vi "AlliGator FLI Dataset Loading Core.vi"(4 "Data Description":string, 5 "Control References":T4, 6 "Metadata":string, 7 "Image Type":string, 8 "error in (no error)":errorcluster, 9 "FLI Data File Information":T1, 10 "selected path":path, 11 "Data Value Reference in":refnum<data-value>) -> (0 "error out":errorcluster, 2 "Message":string, 3 "Data Value Reference out":refnum<data-value>)   [LabVIEW 2021, in "AlliGator Files.lvlib"]
doc: "Core VI handling loading the multiple gate images of a dataset as well as associated information and metadata. It dynamically calls a dataset-specific set of VIs to perform the actual loading."
uses:
  AlliGator Files.lvlib
  GUI/AlliGator Dataset Ctrl Refnums.ctl
  Source Image/AlliGator Displayed Image.ctl
  HDF5/AlliGator FLI Data File Information.ctl
  Phasor/Phasor Fluorescence Lifetime Parameters v3.ctl
  AlliGator FLI Dataset Type.ctl
  Internal Variables/AlliGator Internal Variables v2.ctl
  <vilib>/vision/Image Controls.llb/IMAQ Image.ctl
  Internal Variables/AlliGator Gate Image Set.ctl
  AlliGator Data Series Type.ctl
  Dual-Channel Datasets/AlliGator Dataset Channel.ctl
  Settings/AlliGator Gate Arithmetic.ctl
  Image/Named ROI Description.ctl
  Phasor Graph/AlliGator Decay Metadata v3.ctl
  Decay Analysis/Decay Preprocessing/AlliGator Decay Background Subtraction Info.ctl
  Decay Analysis/Decay Preprocessing/AlliGator Baseline Subtraction Method.ctl
  Graphs/XY Graph/XY Graph Plot Shift Parameters.ctl
  Graphs/XY Graph/XY Graph Plot Shift Method.ctl
  Decay Analysis/Decay Preprocessing/AlliGator Decay Extrapolation Parameters.ctl
  Phasor/Calibration Phasor (m, phi).ctl
  Phasor/Phasor Reference Series.ctl
  Phasor/Phasor Calibration Map v2.ctl
  Phasor/Phasor (g, s).ctl
  Phasor Graph/AlliGator Raw Phasor Plot Data v5.ctl
  Phasor/Phasor Standard Deviation Options.ctl
  Phasor Plot/AlliGator Phasor Multi-Harmonic Data.ctl
  Phasor/Phasor Harmonic Data.ctl
  Decay Fit Parameter Map/AlliGator Decay Fit Options & Parameters v4.ctl
  Fits/IRF(X)PSED/Decay Fit Options v4.ctl
  Fits/Decay Convolution/Decay Model.ctl
  Fits/Residual Type.ctl
  Fits/IRF(X)PSED/Fit Weights Type v2.ctl
  Fits/Non-linear Fitting Method v2.ctl
  Fits/Fit Calculation Method.ctl
  Fits/Non-linear Fitting Algorithm.ctl
  Decay Analysis/Decay Fit/AlliGator Decay Fit Parameter Constraints 2.ctl
  Fits/IRF(X)PSED/Decay Fit Parameters In List.ctl
  Fits/IRF(X)PSED/MLE Baseline Offset Type.ctl
  Decay Analysis/Decay Preprocessing/AlliGator Decay Preprocessing Parameters.ctl
  Fits/IRF(X)PSED/Decay Fit Parameters & Derived Quantities List v2.ctl
  Fits/IRF(X)PSED/Decay Fit Result Constraint.ctl
  Decay Fit Parameter Map/AlliGator Parameter Maps Data.ctl
  AlliGator Image Pre-processing Parameters.ctl
  Arrays/Kernel Type.ctl
  Arrays/Smoothing Algorithm.ctl
  SwissSPAD/SwissSPAD Live_Image Display Options.ctl
  AlliGator Image Pre-processing Step.ctl
  HDF5/AlliGator FLI Image Stack Action.ctl
  Globals, Variables, Constants/AlliGator Variables List.ctl
  AlliGator After Loading Dataset Information.ctl
  AlliGator ICCD-specific Information.ctl
  Globals, Variables, Constants/AlliGator Abort.vi
  <vilib>/Utility/error.llb/Error Cluster From Error Code.vi
  <vilib>/ErrorRing/Error Ring.xnode
  Source Image/AlliGator Source Image.lvlib
  HDF5/AlliGator HDF5.lvlib
  Time/Time.lvlib
  Arrays/Arrays.lvlib
  Strings/Strings.lvlib
  GUI/AlliGator GUI.lvlib
  GUI/GUI.lvlib
  Error/Error.lvlib
  Dual-Channel Datasets/AlliGator Dual-Channel Datasets.lvlib
  Image/Image.lvlib
  SwissSPAD/SwissSPAD Live.lvlib
  Globals, Variables, Constants/AlliGator Globals, Variables & Constants.lvlib
  Files/Files.lvlib
  Phasor/Phasor.lvlib
  Decay Analysis/Decay Preprocessing/AlliGator Decay Preprocessing.lvlib
  Graphs/XY Graph/XY Graph Add-Ons.lvlib
  Phasor Graph/AlliGator Phasor Graph.lvlib
  Phasor Plot/AlliGator Phasor Plot.lvlib
  Fits/Fits.lvlib
  Decay Analysis/Decay Fit/AlliGator Decay Fit.lvlib
  Internal Variables/AlliGator Internal Variables.lvlib
  Settings/AlliGator Settings.lvlib
  Decay Fit Parameter Map/AlliGator Decay Fit Parameter Map.lvlib
panel:
  out "Dual-Channel Dataset":bool
  out "# created images":i32
  out "# Disposed Images":i32
  # "see the AlliGator License on the block diagram (Ctrl+E or Window:Show Block Diagram)"
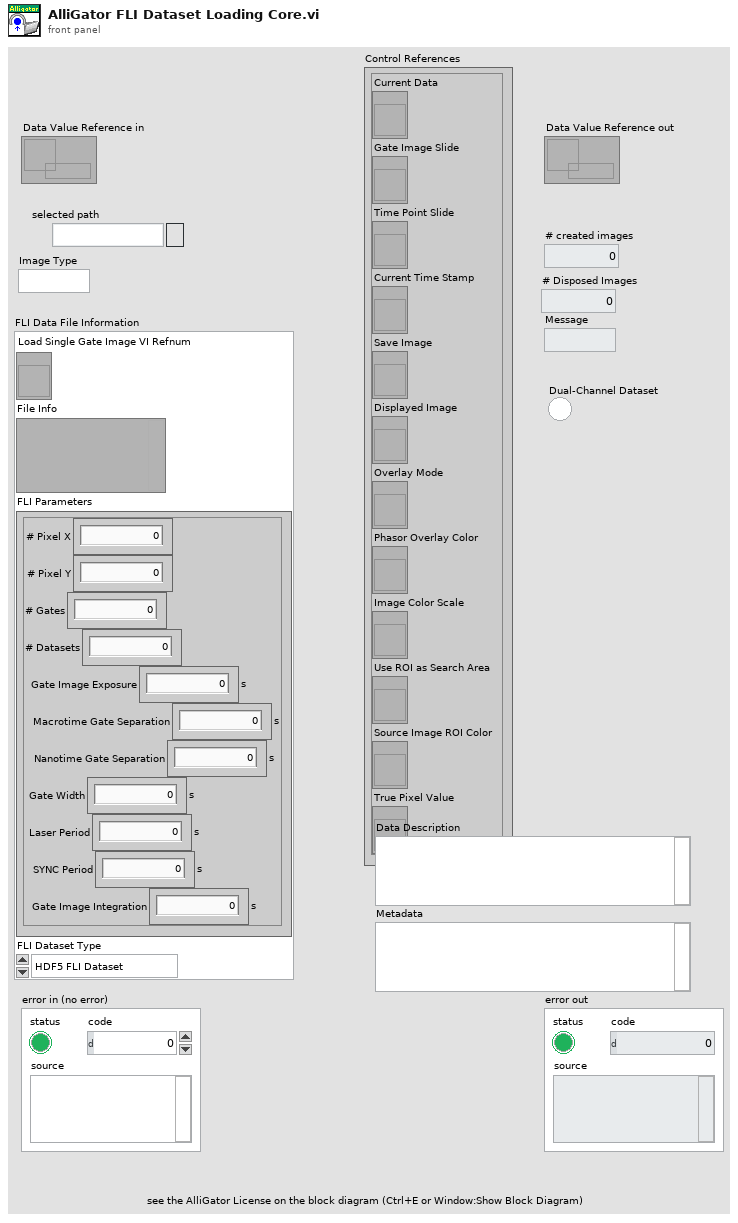
[diagram p1: front panel]
types:
  T1 = typedef "AlliGator HDF5.lvlib/AlliGator FLI Data File Information.ctl" = cluster{"Load Single Gate Image VI Refnum":refnum<vi>, "File Info":variant, "FLI Parameters":T2, "FLI Dataset Type":T3}
  T2 = typedef "Phasor.lvlib/Phasor Fluorescence Lifetime Parameters v3.ctl" = cluster{"# Pixel X":i32, "# Pixel Y":i32, "# Gates":i32, "# Datasets":i32, "Gate Image Exposure":dbl[unit], "Macrotime Gate Separation":dbl[unit], "Nanotime Gate Separation":dbl[unit], "Gate Width":dbl[unit], "Laser Period":dbl[unit], "SYNC Period":dbl[unit], "Gate Image Integration":dbl[unit]}
  T3 = typedef "AlliGator Files.lvlib/AlliGator FLI Dataset Type.ctl" = enum16{"HDF5 FLI Dataset", "Gate Image Folder", ".sdt FLI Dataset (Becker & Hickl)", ".ptu FLI Dataset (PicoQuant)", "SS1 FLI Dataset", "SS2 FLI Dataset", "I/m/phi Dataset", ".bin FLI Dataset (PicoQuant Binned)", ".bin FLI Dataset (Piccolo Binned)", ".mat FLI Dataset"}
  T4 = typedef "AlliGator GUI.lvlib/AlliGator Dataset Ctrl Refnums.ctl" = cluster{"Current Data":refnum<vi>, "Gate Image Slide":refnum<vi>, "Time Point Slide":refnum<vi>, "Current Time Stamp":refnum<vi>, "Save Image":refnum<vi>, "Displayed Image":refnum<vi>, "Overlay Mode":refnum<vi>, "Phasor Overlay Color":refnum<vi>, "Image Color Scale":refnum<vi>, "Use ROI as Search Area":refnum<vi>, "Source Image ROI Color":refnum<vi>, "True Pixel Value":refnum<vi>}
  T5 = typedef "AlliGator Files.lvlib/AlliGator Image Pre-processing Parameters.ctl" = cluster{"Pile-up Correction":bool, "Pixel Well Capacity":u32, "Use Image Binning":bool, "X Bin":i32, "Y Bin":i32, "Use Image Smoothing":bool, "Kernel Type":T6, "Bin":i32, "Algorithm":T7, "Hot Pixel Removal":T8, "Dataset Scaling Factor":dbl, "Image Pre-processing Steps":T9[]}
  T6 = typedef "Arrays.lvlib/Kernel Type.ctl" = enum16{"Uniform", "Bilinear", "Gaussian"}
  T7 = typedef "Arrays.lvlib/Smoothing Algorithm.ctl" = enum16{"Rapid", "Thorough"}
  T8 = typedef "SwissSPAD Live.lvlib/SwissSPAD Live_Image Display Options.ctl" = cluster{"Remove Screamers":bool, "Delta":sgl, "Equalize Histogram":bool, "Percentile":sgl, "Hot Pixel Mask Image":path, "Use Hot Pixel Mask":bool}
  T9 = typedef "AlliGator Files.lvlib/AlliGator Image Pre-processing Step.ctl" = enum16{"Remove Screamers", "Pile-up Correction", "Binning", "Smoothing", "Rescaling", "Dead Left Column Correction"}
  T10 = typedef "AlliGator Source Image.lvlib/AlliGator Image Loading Options.ctl" = cluster{"Pixel Well Capacity":u32, "Pile-up Correction":bool, "Gate Step":i32, "Image Smoothing Options":T11, "Gates to Skip":T12, "File Background Subtraction":bool, "Background File Path":path, "Image Binning Options":T13, "# Gates":u32, "Gates to Keep":T14, "Define Gates to":bool, "Hot Pixel Removal":T8, "Dataset Scaling Factor":dbl, "Image Pre-processing Steps":T9[]}
  T11 = typedef "AlliGator Settings.lvlib/AlliGator Image Smoothing Options.ctl" = cluster{"Use Image Smoothing":bool, "Kernel Type":T6, "Bin":i32, "Algorithm":T7}
  T12 = typedef "AlliGator Settings.lvlib/AlliGator Background Subtraction Parameters.ctl" = cluster{"Start":u32, "End":u32}
  T13 = typedef "AlliGator Source Image.lvlib/AlliGator Image Binning Options.ctl" = cluster{"Use Image Binning":bool, "X Bin":i32, "Y Bin":i32}
  T14 = typedef "AlliGator Settings.lvlib/AlliGator Gates to Keep.ctl" = cluster{"First":u32, "Last":u32}
  T15 = typedef "AlliGator Settings.lvlib/AlliGator Gate Arithmetic.ctl" = enum16{"None", "INT-G2", "G2/INT*<INT>", "(1 - G2/INT)*<INT>"}
  T16 = typedef "AlliGator Dual-Channel Datasets.lvlib/AlliGator Dataset Channel.ctl" = enum16{"G2", "INT"}
  T17 = typedef "Image.lvlib/Image Characteristics.ctl" = cluster{"Calibration":T18, "File Type":string, "X Resolution":i32, "Y Resolution":i32, "File Data Type":i32, "Image Type":T20}
  T18 = typedef "Simple Grid Descriptor" = cluster{"X Step":sgl, "Y Step":sgl, "Unit":T19}
  T19 = typedef "Image Unit" = enum32{"Undefined", "Angström", "Micrometer", "Millimeter", "Centimeter", "Meter", "Kilometer", "Microinch", "Inch", "Feet", "Nautical miles", "Standard miles", "Steps"}
  T20 = typedef "Image Type" = u32
  T21 = typedef "AlliGator HDF5.lvlib/AlliGator FLI Image Stack Action.ctl" = enum16{"Init", "Get Image", "Close"}
  T22 = typedef "AlliGator Globals, Variables & Constants.lvlib/AlliGator Variables List.ctl" = enum16{"---- GUI ----", "GUI:Initialization Status", "GUI:State Indicators Refnum", "GUI:Original AlliGator Menu Items", "GUI:Current Action Loop State", "GUI:Script in progress", "GUI:Playback", "GUI:Loop Playback", "GUI:Search ROI Used", "GUI:Search ROI", "Decay Graph Max Legend Size", "Intensity Graph Max Legend Size", "Decay Statistics Graph Max Legend Size", "Phasor Graph Max Legend Size", "Phasor Ratio Graph Max Legend Size", "Lifetime Graph Max Legend Size", "---- Files ----", "Files:Export Dataset Frames as Individual Files", "Files:Show Batch Export Help Balloons", "Files:Frames in Dataset", "Files:ptu File Frame Start Indices", "Files:Current Frame in Dataset", "Files:Current Frame Timestamp", "Files:Dataset Loaded", "Files:Dataset Metadata", "Files:Dataset Channel", "Files:Dataset Data Description", "Files:Background Dataset Metadata", "Files:Background Dataset Channel", "Files:Background Dataset Data Description", "Files:Background File Subtraction", "Files:Background File Path", "Files:Background File Pile-up Correction", "Files:Background File Pixel Well Capacity", "Files:Background File Scaling Factor", "Files:Current Dataset Load Settings", "Files:Dataset Path", "Files:ICCD-specific Information", "Files:Macrotime Gate Separation", "------ Python Plugins ------", "Python Plugins:Information", "Python Plugins:Python Session", "Python Plugins:Valid Python Session?", "---- Source Image ----", "Source Image:ROIs", "Source Image:Current ROI", "Source Image:ROI Event Refnum", "X_Source Image:Display Range", "X_Source Image:Palette Information", "X_Source Image:Type of Displayed Image", "X_Time Gate Slider", "Source Image:Palette List", "Source Image:Scale", "Source Image:ROI Overlay Color", "Source Image:Overlay to Erase", "Source Image:Is Displayed Image Accumulated", "Source Image:White Light Image Modified", "Source Image:Mask Image Modified", "---- Image Profile Window ----", "Image Profile:Window Event Refnum", "Image Profile:IntensityType", "Image Profile:Intensity Average Type", "Image Profile:Intensity-weighted SDV", "Image Profile:Box Profile Type", "Image Profile:Window Open", "Image Profile:Plotted Fit Parameter", "------ Phasor Graph -------", "Phasor Graph:Show Line", "---- Phasor Plot ---", "Phasor Plot:Parameters Changed", "Phasor Plot:FLI Dataset Modified since last Calculation", "Phasor Harmonics Data", "Selected Phasor Harmonics", "Phasor Harmonic Manager Event Refnum", "Phasor Plot:ROIs", "Phasor Plot:Current ROI", "Phasor Plot:ROI Event Refnum", "Phasor Plot:Image Reference Points", "Phasor Plot:Computed", "Phasor Plot:Palette Information", "Phasor Plot:Palette List", "Phasor Plot:Phasor Ratio Palette Information", "Phasor Plot:Phasor Ratio Palette List", "Phasor Plot:Image Scale", "Phasor Plot:Image Overlay to Erase", "Phasor Plot:Image Elements to Update", "Phasor Plot:Current Calculation Parameters", "Phasor Plot:Current Calibration Options", "Phasor Plot:Reset Cumulated Phasor Plot", "Phasor Plot:Reference 1", "Phasor Plot:Lifetime Reference 1", "Phasor Plot:Reference 1 Frequency", "Phasor Plot:Reference 2", "Phasor Plot:Lifetime Reference 2", "Phasor Plot:Reference 2 Frequency", "---- Decay Analysis ----", "Number of Selected Decays to Fit", "LS Fit Results", "LAR Fit Results", "BS Fit Results", "Last Decay Max - Min", "Best Fit Parameters", "Best Fit Parameter Names", "Actual Size X", "Actual Size Y", "Binning X", "Binning Y", "Actual # Gates", "Dataset Number", "Gates to...", "Gates Skipped", "Gates to keep", "Gate Step", "Gate Separation", "Reversed Gates", "Pile-up Correction", "Pixel Well Capacity", "Background Subtracted", "Background Subtraction Method", "Background Definition Range", "Background File (deprecated)", "Number of Dataset Accumulated", "Array of Accumulated Dataset Paths", "Do Averaged Datasets", "Destination File Path", "Process Plot Target", "Use 1/D as Phasor Frequency", "---- Decay Fit Parameter Map -----", "Decay Fit Parameter Map:Palette Information", "Decay Fit Parameter Map:Palette List", "Decay Fit Parameter Map:X Resolution", "Decay Fit Parameter Map:Y Resolution", "Decay Fit Parameter Map:Use Decay Fit Result Constraints", "Decay Fit Parameter Map:Decay Fit Result Constraints", "Decay Fit Parameter Map:Decay Fit Result Constraints Applied", "---- Parameter Map ----", "Parameter Map:Palette Information", "Parameter Map:Palette List", "------- Local Decay Window ---------", "Local Decay Graph Window:Event Refnum", "Local Decay Graph Window:Use normalized IRF for convolution", "----- Miscellaneous ----", "Misc:Skippable Dialog Windows Status"}
  T23 = typedef "AlliGator Internal Variables.lvlib/AlliGator Internal Variables v2.ctl" = cluster{"----------------------------- Images -----------------------------":u8, "Displayed Image":T24, "White Light Image":T24, "Mask Image":T24, "ROI Mask Image":T24, "Current Dataset Images 1":T25, "Background Dataset Images 1":T25, "Current Dataset Images 2":T25, "Background Dataset Images 2":T25, "Current Dataset Arithmetic Images":T25, "Accumulated Dataset Images 1":T25, "Accumulated Dataset Images 2":T25, "Accumulated Dataset Arithmetic Images":T25, "----------------------------- File Paths -----------------------------":u8, "Phasor Plot Image":T24, "Decay Fit Parameter Map Image":T24, "Parameter Map Image":T24, "Single Data Point Path":path, "White Light Image Path":path, "Mask Image Path":path, "Time-Series Folder":path, "[Time-Series Paths]":path[], "----------------------------- FLI Dataset -----------------------------":u8, "Current Dataset":i32, "Single Dataset Type":T3, "Current Folder":string, "AlliGator Data Series Type":T26, "# Datasets":i32, "Dual-Channel Dataset":bool, "Selected Channel Name":string, "Dataset Channel":T16, "Channel Arithmetic":T15, "Dual-Channel Background Dataset":bool, "Background Channel":T16, "Dual-Channel Accumulated Dataset":bool, "Start Time":dbl, "[Time-Series Timestamps]":dbl[], "[Intensity Corrections]":dbl[], "Time Series Script":bool, "Type of Displayed Image":T27, "Gate Image Slide":u16, "# Gates":i32, "ROIs":T28[], "----------------------------- Decays -----------------------------":u8, "ROI Decay":cluster{"t Array":dbl[], "I Array":dbl[]}, "Valid Decay":bool, "Decay  Metadata":T30, "Reference Decay Plot Name":string, "Reference Decay":cluster{"t Array":dbl[], "I Array":dbl[]}, "Decay Shift Plot":cluster{"Time Stamps":dbl[], "Decay Shifts":dbl[]}, "[Decays Max Values]":sgl[], "[Decays Min Values]":sgl[], "----------------------------- Calibration -----------------------------":u8, "Calibration Phasor":T36, "Calibration Phasor Series":T37, "Phasor Calibration Map":T38, "Calibration Map MD5 Digest":string, "----------------------------- Phasor Graph -----------------------------":u8, "Last Raw Phasor":T39, "Last Calibrated Phasor":T39, "Last Calibrated Phasor SDV":T39, "Phasor Graph:Phasor Plot":cluster{"g Array":dbl[], "s Array":dbl[]}, "Phasor Graph:Phasor SDV Plot":cluster{"g Array":dbl[], "s Array":dbl[]}, "[Phasor Graph:Raw Phasor Plots]":T40[], "Phasor Plot locked to Ref 1":i32, "[Phasor Plot(s) locked to Ref 1]":i32[], "[Phasor Plot(s) locked to Ref 2]":i32[], "[Pixel Phasors]":T39[], "----------------------------- Phasor Plot -----------------------------":u8, "[[Sum Image]]":dbl[][], "[[CSG Phasors]]":csg[][], "[[Valid Pixel?]]":bool[][], "[[Phasor Ratios]]":dbl[][], "[[Average Lifetimes]]":dbl[][], "Amplitude Weighted Average Lifetime":bool, "I/m/phi Dataset":cluster{"I/m/phi Dataset?":bool, "Base Frequency":dbl[unit], "Harmonic Orders":u8[]}, "Multi Phasor Plot Data":T42, "----------------------------- Decay Fit Parameter Map -----------------------------":u8, "Decay Fit Options & Parameters":T44, "Fit Options: Decay Preprocessing Parameters":T55, "Fit Options: Reference Decay":cluster{"t Array":dbl[], "I Array":dbl[]}, "Is Full Image Parameters Map":bool, "Is Single-Pixels Parameters Map":bool, "NLSF Parameters Map X Resolution":i32, "NLSF Parameters Map Y Resolution":i32, "[Single Decay Fit Parameters]":dbl[], "Fit Model":T46, "[[Multiple Decays Fit Parameters]]":dbl[][], "[[Multiple Decays Fit Parameter SDVs]]":dbl[][], "[[IRFs]]":dbl[][], "[ROI Descriptors]":T29[], "IRF Array Time Axis":dbl[], "Decay Array Time Axis":dbl[], "[Decay Fit Parameter Names]":T56[], "[Decay Sum]":dbl[], "Array of Decay Fit Result Constraints":T57[], "Selected ROIs Array":bool[], "----------------------------- Parameter Maps -----------------------------":u8, "[Map Set Names]":string[], "[Parameter Maps]":T58[], "[[User-defined Quantities]]":dbl[][], "User-defined Quantity":string}
  T24 = typedef "IMAQ Image.ctl" = refnum<image>
  T25 = typedef "AlliGator Internal Variables.lvlib/AlliGator Gate Image Set.ctl" = cluster{"SGL Image Max":T24, "SGL Image Sum":T24, "SGL Gate Images":T24[], "SGL Image Min":T24}
  T26 = typedef "AlliGator Files.lvlib/AlliGator Data Series Type.ctl" = enum16{"Not a Supported Series", "Gate Images Folder Series", "SwissSPAD 2 Dataset Series", "B&H FLI Dataset Series", "PicoQuant PTU FLI Dataset Series", "PicoQuant BIN FLI Dataset Series", "Piccolo hist BIN FLI Dataset Series", "HDF5 FLI Dataset Series"}
  T27 = typedef "AlliGator Source Image.lvlib/AlliGator Displayed Image.ctl" = enum16{"Single Gate", "Sum of All Gates", "Max of All Gates", "Min of All Gates", "-", "White Ligth Image", "Mask Image"}
  T28 = typedef "Image.lvlib/Named ROI Description.ctl" = cluster{"ROI Descriptor":T29, "ROI Name":string, "Overlay Color":u32}
  T29 = typedef "ROI Descriptor" = cluster{"Global Rectangle":i32[], "Contours":cluster{"ID":enum32{"External", "Internal"}, "Type":u32, "Coordinates":i32[]}[]}
  T30 = typedef "AlliGator Phasor Graph.lvlib/AlliGator Decay Metadata v3.ctl" = cluster{"ROI Descriptor":T29, "ROI Center":cluster{"X":i32, "Y":i32}, "Decay Background Subtraction Info":T31, "Decay Reverted":bool, "Decay Smoothened":bool, "Decay Straightened":bool, "Fitted Tau (Decay Straightening)":dbl, "Decay Shift Parameters":T33, "Decay Shifted":bool, "Decay Extrapolated":bool, "Decay Extrapolation Parameters":T35, "Decay Normalized":bool, "Fold Decay":bool, "# Folds":u32}
  T31 = typedef "AlliGator Decay Preprocessing.lvlib/AlliGator Decay Background Subtraction Info.ctl" = cluster{"Laser Period":dbl[unit], "Gate Duration":dbl[unit], "Baseline Subtraction Method":T32, "Background Definition Range":cluster{"Min Gate":dbl[unit], "Max Gate":dbl[unit]}, "Total Intensity w/o Bkgd Subtraction":dbl, "Bkgd-subtracted Intensity (exp)":dbl, "# Data Points":i32, "Background/Gate":dbl, "Fitted Lifetime":dbl[unit], "Bkgd-subtracted Intensity (theo)":dbl}
  T32 = typedef "AlliGator Decay Preprocessing.lvlib/AlliGator Baseline Subtraction Method.ctl" = enum16{"Mean", "Min", "Square Gated Single-Exponential", "File", "Constant"}
  T33 = typedef "XY Graph Add-Ons.lvlib/XY Graph Plot Shift Parameters.ctl" = cluster{"Type":T34, "Shift":dbl[unit], "Threshold":dbl, "Rotate":bool}
  T34 = typedef "XY Graph Add-Ons.lvlib/XY Graph Plot Shift Method.ctl" = enum16{"Default", "CFD", "Threshold", "Cross-Correlation"}
  T35 = typedef "AlliGator Decay Preprocessing.lvlib/AlliGator Decay Extrapolation Parameters.ctl" = cluster{"Additional Points":u32, "Head Fraction":dbl, "Fitted Tau":dbl, "Use Periodicity":bool, "Use Cursors":bool, "Tail Fraction":dbl}
  T36 = typedef "Phasor.lvlib/Calibration Phasor (m, phi).ctl" = cluster{"m":dbl, "phi":dbl, "Phasor Frequency":dbl[unit], "Reference Lifetime":dbl[unit]}
  T37 = typedef "Phasor.lvlib/Phasor Reference Series.ctl" = cluster{"m Array":dbl[], "phi Array":dbl[], "Phasor Frequency":dbl[unit], "Calibration Lifetime":dbl[unit]}
  T38 = typedef "Phasor.lvlib/Phasor Calibration Map v2.ctl" = cluster{"Phasor Frequency":dbl[unit], "Calibration Lifetime":dbl[unit], "ROI Centers":cluster{"X":i32, "Y":i32}[], "ROI Descriptors":T29[], "Map Resolution X":i32, "Map Resolution Y":i32, "z Array":cdb[]}
  T39 = typedef "Phasor.lvlib/Phasor (g, s).ctl" = cluster{"g":dbl, "s":dbl}
  T40 = typedef "AlliGator Phasor Graph.lvlib/AlliGator Raw Phasor Plot Data v5.ctl" = cluster{"Phasor Plot Name":string, "Raw Phasor Plot":T39[], "Phasor Frequency":dbl[unit], "[Decay Metadata]":T30[], "Raw Phasor Plot SDV":T39[], "Phasor SDV Options":T41, "[Calibration Phasor]":T36[], "Intensity Array":dbl[]}
  T41 = typedef "Phasor.lvlib/Phasor Standard Deviation Options.ctl" = cluster{"Compute Estimated SDV":bool, "# Replicas":u32, "Use Estimated Average Phasor":bool}
  T42 = typedef "AlliGator Phasor Plot.lvlib/AlliGator Phasor Multi-Harmonic Data.ctl" = cluster{"Base Frequency":dbl[unit], "# Harmonics":u8, "Harmonic Orders":u8[], "Phasor Plot Settings Checksum":u64, "Phasor Harmonic Data Array":T43[]}
  T43 = typedef "Phasor.lvlib/Phasor Harmonic Data.ctl" = cluster{"Phasor Harmonic Name":string, "Phasor Plot Settings Checksum":u64, "Phasor Frequency":dbl[unit], "Base Frequency":dbl[unit], "Harmonic Order":u8, "Phasor Plot Parameters":string, "Phasor Array [[CSG]]":csg[][], "Dataset File Path":path}
  T44 = typedef "AlliGator Decay Fit Parameter Map.lvlib/AlliGator Decay Fit Options & Parameters v4.ctl" = cluster{"SYNC Period":dbl[unit], "Fit Options":T45, "Fit Parameter Constraints":T52[], "MLE Baseline Offset":dbl, "MLE Baseline Offset Type":T54}
  T45 = typedef "Fits.lvlib/Decay Fit Options v4.ctl" = cluster{"Show Fit Residuals":bool, "Fit Model":T46, "Residual Type":T47, "Max Decay Percentile":dbl, "Min Decay Percentile":dbl, "Show Full Decay":bool, "Weights":T48, "Fitting Method":T49, "Compute Parameter Uncertainties":bool, "Periodic Boundaries":bool, "Model Calculation":T50, "Period":dbl[unit], "Termination Criteria":cluster{"Max Iterations":i32, "Max Function Calls":i32, "Max Time":dbl[unit], "Function Tolerance":dbl, "Parameter Tolerance":dbl, "Gradient Tolerance":dbl, "Min Lambda":dbl, "Max Lambda":dbl, "Initial Tick Count":u32}, "Offset Resolution":dbl[unit], "Use Local IRF":bool, "Fitting Algorithm":T51, "Show Confidence Interval ":bool, "Confidence Level":dbl}
  T46 = typedef "Fits.lvlib/Decay Model.ctl" = enum16{"1-Exponential", "2-Exponentials"}
  T47 = typedef "Fits.lvlib/Residual Type.ctl" = enum16{"Standard", "Normalized", "Reduced"}
  T48 = typedef "Fits.lvlib/Fit Weights Type v2.ctl" = enum16{"Unweighted", "1/Variance (Neyman)", "1/Variance (Pearson)", "Best of All"}
  T49 = typedef "Fits.lvlib/Non-linear Fitting Method v2.ctl" = enum16{"Least Square", "Least Absolute Residual", "Bisquare", "MLE", "-", "Best of All"}
  T50 = typedef "Fits.lvlib/Fit Calculation Method.ctl" = enum16{"Simulation", "Convolution", "Integration"}
  T51 = typedef "Fits.lvlib/Non-linear Fitting Algorithm.ctl" = enum16{"Levenberg-Marquardt", "Trust-Region Dogleg"}
  T52 = typedef "AlliGator Decay Fit.lvlib/AlliGator Decay Fit Parameter Constraints 2.ctl" = cluster{"Fit Parameter":T53, "Min Value":dbl, "Max Value":dbl, "Global":bool, "Used":bool}
  T53 = typedef "Fits.lvlib/Decay Fit Parameters In List.ctl" = enum16{"Offset", "Baseline", "A_1", "tau_1", "A_2", "tau_2"}
  T54 = typedef "Fits.lvlib/MLE Baseline Offset Type.ctl" = enum32{"Absolute", "Percentage"}
  T55 = typedef "AlliGator Decay Preprocessing.lvlib/AlliGator Decay Preprocessing Parameters.ctl" = cluster{"Background Subtraction":bool, "Straighten Decay":bool, "Reverse Gates":bool, "1-Normalized Decay":bool, "Smoothen Decay":bool, "Smoothing Parameter":dbl, "Shift Decay":bool, "Decay Shift Parameters":T33, "Extrapolate Decay":bool, "Additional Points":u32, "Head Fraction":dbl, "Pixel-Normalize Decay":bool, "Use Periodicity":bool, "Use Cursors":bool, "Tail Fraction":dbl, "Use Decay Pre-Processing":bool, "Fold Decay":bool, "# Folds":u32, "[0-1]-Normalized Decay":bool}
  T56 = typedef "Fits.lvlib/Decay Fit Parameters & Derived Quantities List v2.ctl" = enum16{"Offset", "Baseline", "A_1", "tau_1", "A_2", "tau_2", "<tau>_a", "f1_a", "f2_a", "<tau>_i", "f1_i", "f2_i", "-", "R^2", "Chi^2"}
  T57 = typedef "Fits.lvlib/Decay Fit Result Constraint.ctl" = cluster{"Fit Parameter":enum16{"Offset", "Baseline", "A_1", "tau_1", "A_2", "tau_2", "<tau>_a", "f1_a", "f2_a", "<tau>_i", "f1_i", "f2_i", "-", "R^2", "Chi^2", "Max Relative Residual", "<Residual ACF>", "Residual ACF SDV", "tau_2/tau_1"}, "Min Value":dbl, "Max Value":dbl, "Use Constraint":bool}
  T58 = typedef "AlliGator Decay Fit Parameter Map.lvlib/AlliGator Parameter Maps Data.ctl" = cluster{"Map Set Name":string, "[Parameter Names]":string[], "[[Parameters]]":dbl[][], "[[Parameter SDVs]]":dbl[][], "Decay Array Time Axis":dbl[], "[[IRFs]]":dbl[][], "IRF Array Time Axis":dbl[], "X Resolution":i32, "Y Resolution":i32, "Intensity Array":dbl[]}
  T59 = typedef "AlliGator Files.lvlib/AlliGator ICCD-specific Information.ctl" = cluster{"V MCP":dbl[unit], "X Hardware Binning":dbl, "Y Hardware Binning":dbl, "Gate Image Integration":dbl[unit], "Laser Power":dbl[unit]}
  T60 = typedef "AlliGator Files.lvlib/AlliGator After Loading Dataset Information.ctl" = cluster{"Nanotime Gate Separation":dbl[unit], "Gate Width":dbl[unit], "Laser Period":dbl[unit], "Data Description":string, "# Pixel X":i32, "# Pixel Y":i32, "Gates to Use":cluster{"Start":u32, "End":u32}, "Gate Step":i32, "SYNC Period":dbl[unit], "X Binning":i32, "Y Binning":i32, "Gates to":bool, "Metadata":string, "Gate Image Exposure":dbl[unit], "Gate Image Integration":dbl[unit], "Macrotime Gate Separation":dbl[unit], "ICCD-specific Information":T59}
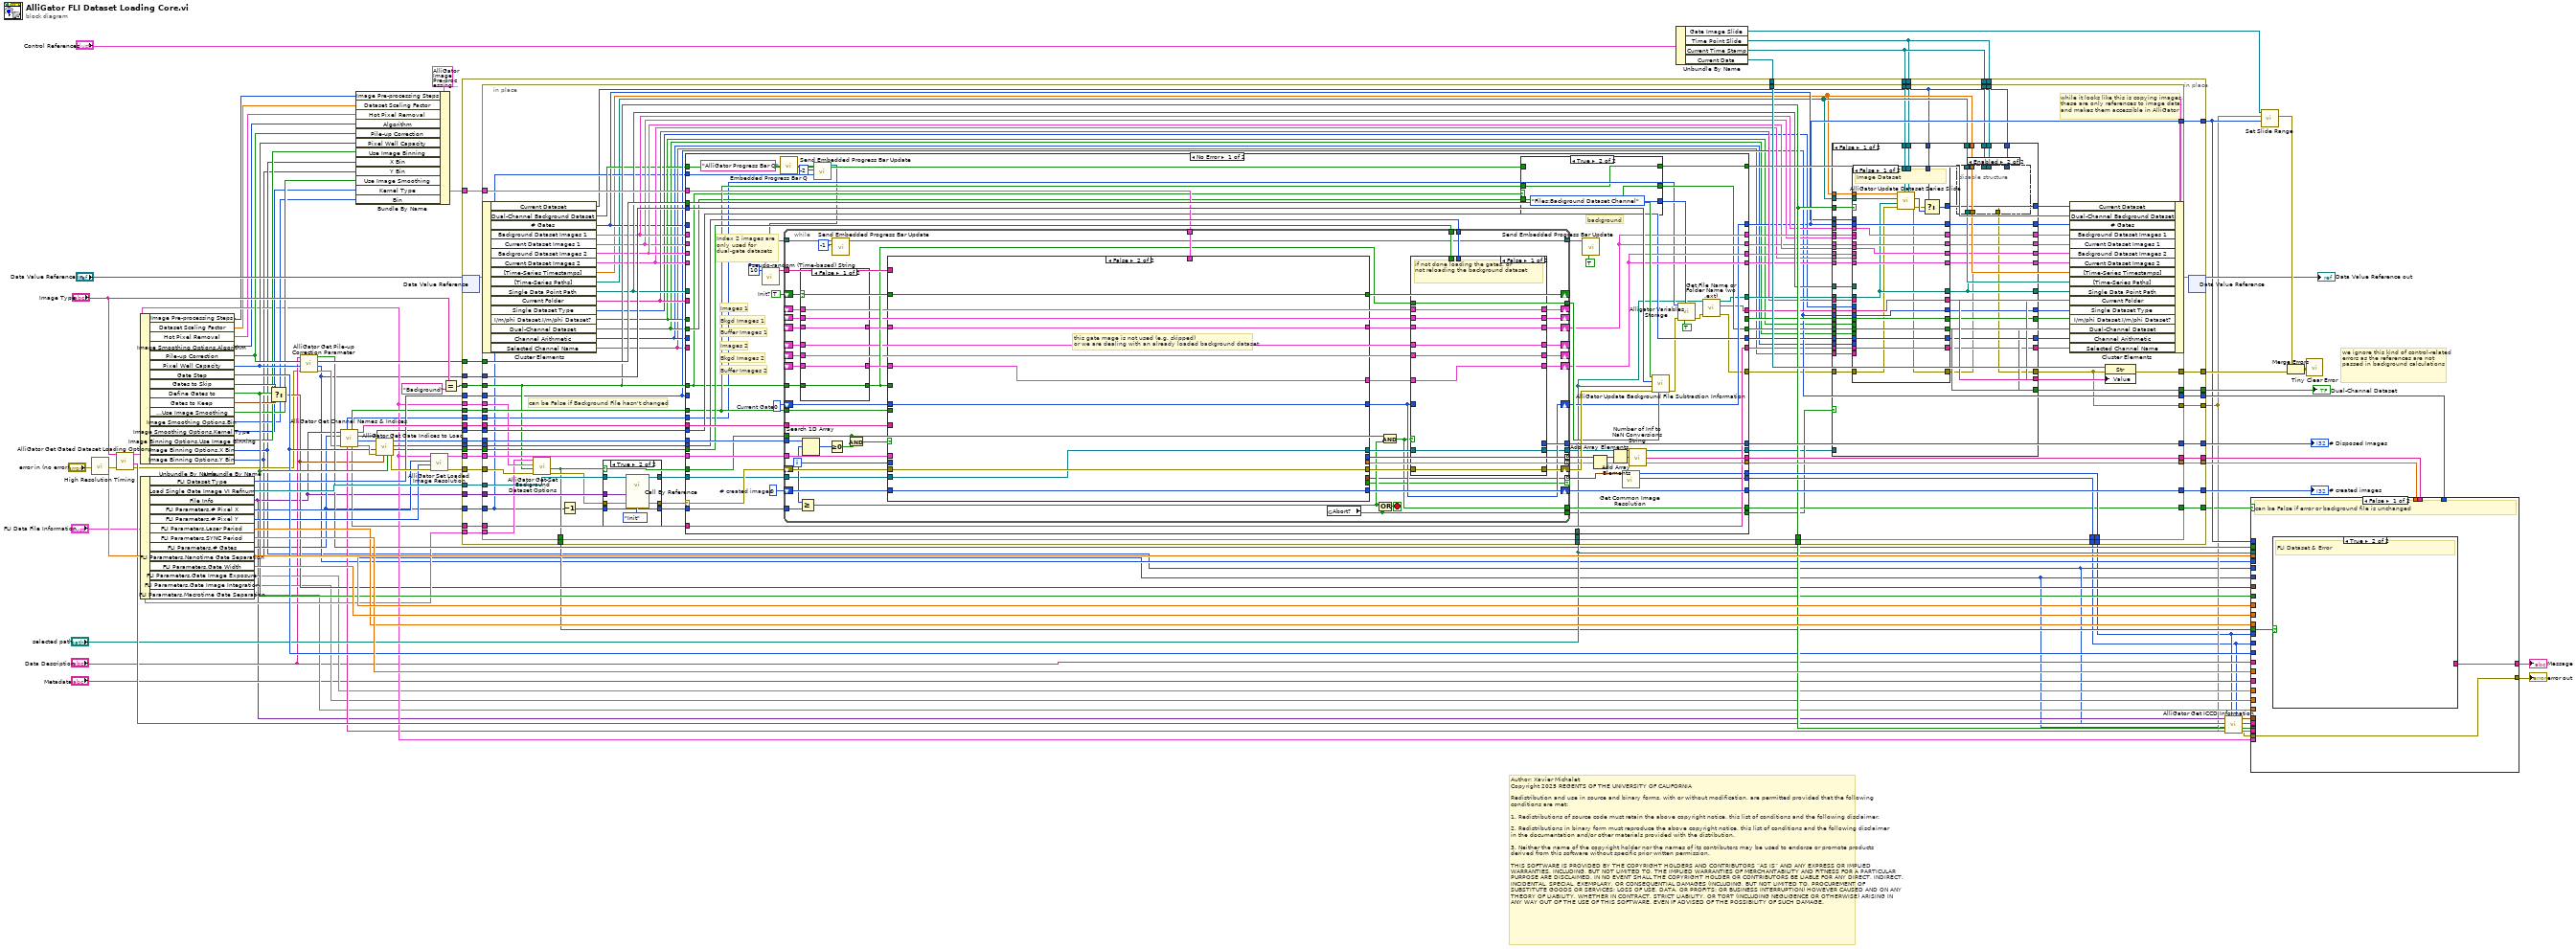
[diagram p0: block diagram]
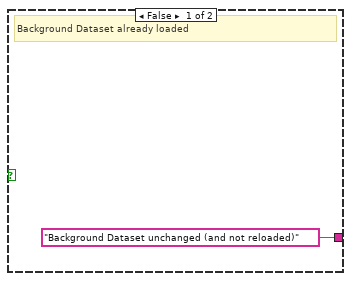
[diagram p2: hidden frame]
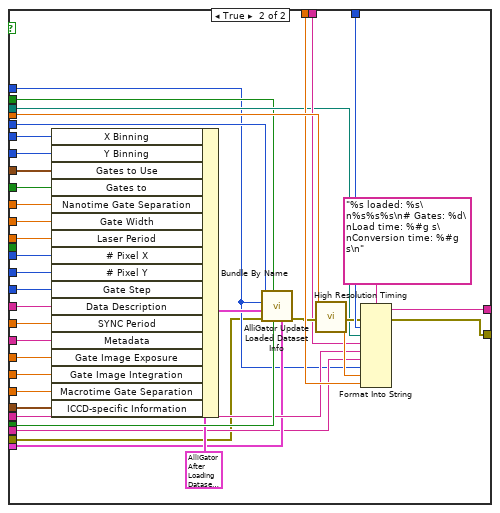
[diagram p3: hidden frame]
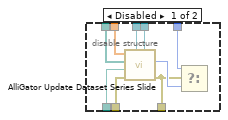
[diagram p4: hidden frame]
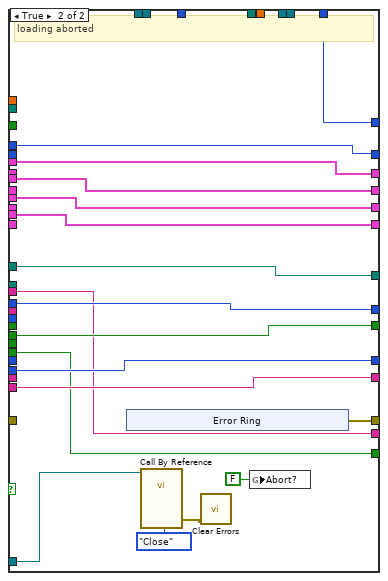
[diagram p6: hidden frame]
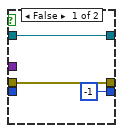
[diagram p7: hidden frame]
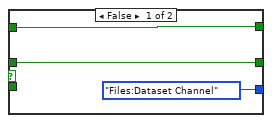
[diagram p8: hidden frame]
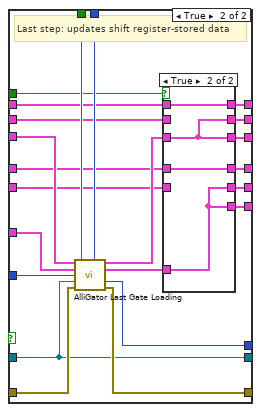
[diagram p9: hidden frame]
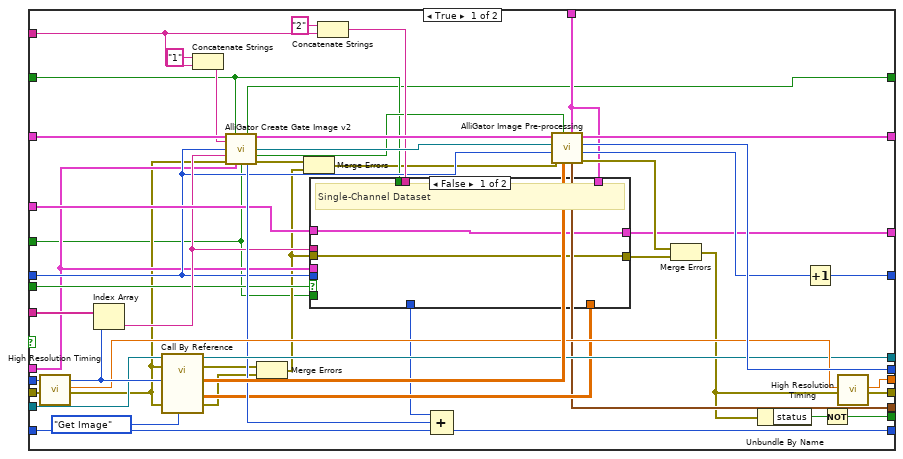
[diagram p11: hidden frame]
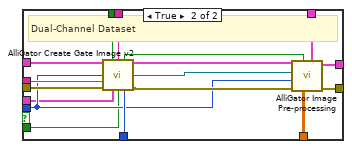
[diagram p12: hidden frame]
diagram:
  # "Author: Xavier Michalet\nCopyright 2025 REGENTS OF THE UNIVERSITY OF CALIFORNIA\n\nRedistribution and use in source and binary forms, with or without modification, are permitted provided that the following conditions are met:\n\n1. Redistributions of source code must retain the above copyright notice, this list of conditions and the following disclaimer.\n\n2. Redistributions in binary form must reproduce the above copyright notice, this list of conditions and the following disclaimer in the documentation and/or other materials provided with the distribution.\n\n3. Neither the name of the copyright holder nor the names of its contributors may be used to endorse or promote products derived from this software without specific prior written permission.\n\nTHIS SOFTWARE IS PROVIDED BY THE COPYRIGHT HOLDERS AND CONTRIBUTORS “AS IS” AND ANY EXPRESS OR IMPLIED WARRANTIES, INCLUDING, BUT NOT LIMITED TO, THE IMPLIED WARRANTIES OF MERCHANTABILITY AND FITNESS FOR A PARTICULAR PURPOSE ARE DISCLAIMED. IN NO EVENT SHALL THE COPYRIGHT HOLDER OR CONTRIBUTORS BE LIABLE FOR ANY DIRECT, INDIRECT, INCIDENTAL, SPECIAL, EXEMPLARY, OR CONSEQUENTIAL DAMAGES (INCLUDING, BUT NOT LIMITED TO, PROCUREMENT OF SUBSTITUTE GOODS OR SERVICES; LOSS OF USE, DATA, OR PROFITS; OR BUSINESS INTERRUPTION) HOWEVER CAUSED AND ON ANY THEORY OF LIABILITY, WHETHER IN CONTRACT, STRICT LIABILITY, OR TORT (INCLUDING NEGLIGENCE OR OTHERWISE) ARISING IN ANY WAY OUT OF THE USE OF THIS SOFTWARE, EVEN IF ADVISED OF THE POSSIBILITY OF SUCH DAMAGE."
  # "we ignore this kind of control-related errors as the references are not passed in background calculations"
  n1 = call "High Resolution Timing.vi"("Error In"="error in (no error)") -> ("elapsed (relative) seconds"=w89:dbl, "Error Out"=w90:errorcluster)  [unwired: 16 in, 1 out]
  n2 = call "AlliGator Get Gated Dataset Loading Options.vi"("error in (no error)"=w90, "Image Type"="Image Type") -> ("error out"=w18:errorcluster, "Dataset Loading Options string"=w52:string, "Dataset Loading Options"=w32:T10)  [unwired: 6 in, 1 out]
  n3 = Unbundle By Name(w32) -> ("Image Pre-processing Steps"=w14:T9[], "Dataset Scaling Factor"=w15:dbl, "Hot Pixel Removal"=w13:T8, "Image Smoothing Options.Algorithm"=w12:T7, "Pile-up Correction"=w43:bool, "Pixel Well Capacity"=w42:u32, "Gate Step"=w65:i32, "Gates to Skip"=w64:T12, "Define Gates to"=w66:bool, "Gates to Keep"=w63:T14, "Image Smoothing Options.Use Image Smoothing"=w40:bool, "Image Smoothing Options.Bin"=w38:i32, "Image Smoothing Options.Kernel Type"=w39:T6, "Image Binning Options.Use Image Binning"=w41:bool, "Image Binning Options.X Bin"=w6:i32, "Image Binning Options.Y Bin"=w5:i32)
  n4 = Unbundle By Name("FLI Data File Information") -> ("FLI Dataset Type"=w80:T3, "Load Single Gate Image VI Refnum"=w77:refnum<vi>, "File Info"=w11:variant, "FLI Parameters.# Pixel X"=w50:i32, "FLI Parameters.# Pixel Y"=w51:i32, "FLI Parameters.Laser Period"=w73:dbl[unit], "FLI Parameters.SYNC Period"=w74:dbl[unit], "FLI Parameters.# Gates"=w16:i32, "FLI Parameters.Nanotime Gate Separation"=w75:dbl[unit], "FLI Parameters.Gate Width"=w76:dbl[unit], "FLI Parameters.Gate Image Exposure"=w27:dbl[unit], "FLI Parameters.Gate Image Integration"=w26:dbl[unit], "FLI Parameters.Macrotime Gate Separation"=w24:dbl[unit])
  n5 = Select(t=w64, s=w66, f=w63) -> (s? t:f=w29:T14)
  n6 = call "AlliGator Get Pile-up Correction Parameter.vi"("error in (no error)"=w18, "Pixel Well Capacity in"=w42, "Pile-up Correction in"=w43, "Data Information"="Data Description") -> ("error out"=w17:errorcluster, "Pixel Well Capacity out"=w7:u32, "Pile-up Correction out"=w46:bool, "Pile-up Correction (already) applied?"=w44:bool)  [unwired: 4 in]
  n7 = call "AlliGator Get Channel Names & Indices.vi"("error in (no error)"=w17, "# Gates"=w16, "File Info"=w11) -> ("error out"=w83:errorcluster, "Gate Indices"=w82:i32[], "Channel Arithmetic"=w34:T15, "Gate Image Names"=w81:string[], "Selected Channel Name"=w28:string, "Dual-Channel Dataset"=w35:bool, "Selected Channel Message"=w30:string, "Dataset Channel"=w25:T16)  [unwired: 1 in]
  n8 = Bundle By Name(cluster=T5 {"Pile-up Correction"=FALSE, "Pixel Well Capacity"=0, "Use Image Binning"=FALSE, "X Bin"=0, "Y Bin"=0, "Use Image Smoothing"=FALSE, "Kernel Type"=enum."Uniform", "Bin"=0, "Algorithm"=enum."Rapid", "Hot Pixel Removal"={"Remove Screamers"=FALSE, "Delta"=0.0, "Equalize Histogram"=FALSE, "Percentile"=0.0, "Hot Pixel Mask Image"=path "", "Use Hot Pixel Mask"=FALSE}, "Dataset Scaling Factor"=0.0, "Image Pre-processing Steps"=[]}, "Image Pre-processing Steps"=w14, "Dataset Scaling Factor"=w15, "Hot Pixel Removal"=w13, "Algorithm"=w12, "Pile-up Correction"=w43, "Pixel Well Capacity"=w42, "Use Image Binning"=w41, "X Bin"=w6, "Y Bin"=w5, "Use Image Smoothing"=w40, "Kernel Type"=w39, "Bin"=w38) -> (w36:T5)
  n9 = call "AlliGator Get Gate Indices to Load.vi"("Gates to?"=w66, "Gates to Use"=w29, "Error In"=w83, "Gate Step"=w65, "Gate Indices in"=w82) -> ("Error Out"=w84:errorcluster, "Gates across boundaries?"=w68:bool, "Split Index"=w67:u32, "Gate Indices out"=w62:i32[])  [unwired: 3 in]
  n10 = call "AlliGator Set Loaded Image Resolution.vi"("Error In"=w84, "Image Y"=w51, "Image X"=w50, "Image Loading Options"=w32) -> ("Error Out"=w53:errorcluster, "Image Characteristics"=w49:T17)  [unwired: 6 in]
  n11 = Equal?(x="Image Type", y="Background" ("x")) -> (x = y?=w70:bool)
  n12 = Unbundle By Name("Control References") -> ("Gate Image Slide"=w56:refnum<vi>, "Time Point Slide"=w1:refnum<vi>, "Current Time Stamp"=w2:refnum<vi>, "Current Data"=w55:refnum<vi>)
  n13 = in-place {
    in-place-border: [w132] -> w85
    in-place-border: w81 -> [w131]
    in-place-border: w62 -> [w130]
    in-place-border: [w129] -> w48
    in-place-border: w49 -> [w128]
    in-place-border: [w127] -> w86
    in-place-border: w16 -> [w126]
    in-place-border: w46 -> [w125]
    in-place-border: [w124] -> w9
    in-place-border: w7 -> [w123]
    in-place-border: w53 -> [w122]
    in-place-border: "selected path" -> [w121]
    in-place-border: w55 -> [w118]
    in-place-border: [w117] -> w21
    in-place-border: [w116] -> w60
    in-place-border: w67 -> [w115]
    in-place-border: w68 -> [w114]
    in-place-border: w70 -> [w113]
    in-place-border: [w112] -> w72
    in-place-border: w11 -> [w111]
    in-place-border: w77 -> [w110]
    in-place-border: [w109] -> w78
    in-place-border: [w108] -> w79
    in-place-border: w80 -> [w107]
    in-place-border: w36 -> [w106]
    in-place-border: w35 -> [w105]
    in-place-border: w34 -> [w104]
    in-place-border: [w103] -> w33
    in-place-border: w32 -> [w102]
    in-place-border: "FLI Data File Information" -> [w101]
    in-place-border: w28 -> [w100]
    in-place-border: [w99] -> w4
    in-place-border: [w98] -> w3
    in-place-border: w25 -> [w97]
    in-place-border: [w96] -> w20
    in-place-border: [w95] -> w19
    in-place-border: w2 -> [w94]
    in-place-border: w1 -> [w93]
    in-place-border: w2 -> [w92]
    in-place-border: w1 -> [w91]
    n14 = in-place-dvr #1("Data Value Reference in") -> (w120:T23)  [unwired: 1 out]
    n15 = in-place {
      in-place-border: [w217] -> w132
      in-place-border: w131 -> [w216]
      in-place-border: w130 -> [w215]
      in-place-border: [w214] -> w129
      in-place-border: w128 -> [w213]
      in-place-border: [w212] -> w127
      in-place-border: w126 -> [w141]
      in-place-border: w125 -> [w211]
      in-place-border: [w140] -> w124
      in-place-border: w123 -> [w210]
      in-place-border: w122 -> [w203]
      in-place-border: w121 -> [w209]
      in-place-border: w118 -> [w208]
      in-place-border: [w156] -> w117
      in-place-border: [w207] -> w116
      in-place-border: w115 -> [w206]
      in-place-border: w114 -> [w205]
      in-place-border: w113 -> [w186]
      in-place-border: [w186] -> w112
      in-place-border: w111 -> [w202]
      in-place-border: w110 -> [w201]
      in-place-border: [w161] -> w109
      in-place-border: [w199] -> w108
      in-place-border: w107 -> [w161]
      in-place-border: w106 -> [w198]
      in-place-border: w105 -> [w194]
      in-place-border: w104 -> [w197]
      in-place-border: [w165] -> w103
      in-place-border: w102 -> [w193]
      in-place-border: w101 -> [w192]
      in-place-border: w100 -> [w191]
      in-place-border: [w190] -> w99
      in-place-border: [w189] -> w98
      in-place-border: w97 -> [w187]
      in-place-border: [w149] -> w96
      in-place-border: [w148] -> w95
      in-place-border: w94 -> [w145]
      in-place-border: w93 -> [w144]
      in-place-border: w92 -> [w135]
      in-place-border: w91 -> [w134]
      # "can be False if Background File hasn't changed"
      # "while it looks like this is copying images,\nthese are only references to image data, \nand makes them accessible in AlliGator"
      n16 = in-place-cluster #2(w120) -> ("Current Dataset"=w133:i32, "Dual-Channel Background Dataset"=w157:bool, "# Gates"=w154:i32, "Background Dataset Images 1"=w180:T25, "Current Dataset Images 1"=w174:T25, "Background Dataset Images 2"=w177:T25, "Current Dataset Images 2"=w171:T25, "[Time-Series Timestamps]"=w136:dbl[], "[Time-Series Paths]"=w137:path[], "Single Data Point Path"=w185:path, "Current Folder"=w181:string, "Single Dataset Type"=w160:T3, "I/m/phi Dataset.I/m/phi Dataset?"=w153:bool, "Dual-Channel Dataset"=w152:bool, "Channel Arithmetic"=w151:T15, "Selected Channel Name"=w150:string)
      n17 = call "AlliGator Get-Set Background Dataset Options.vi"("error in (no error)"=w203, "Background Dataset"=w186, "Image Loading Options"=w193, "FLI Data File Information"=w192) -> ("error out"=w196:errorcluster, "Load Dataset?"=w148:bool)  [unwired: 6 in]
      n18 = Decrement(x=w141) -> (x-1=w142:i32)
      n19 = case shown="True" w148 {
        tunnel: [w337 w344] -> w204
        tunnel: w202 -> [_ w343]
        tunnel: w201 -> [w338 w342]
        tunnel: [w338 w341] -> w200
        tunnel: w196 -> [w337 w340]
        tunnel: w142 -> [_ w339]
        tunnel: [-1 w339] -> w195
        frame False {
        }
        frame True {
          n20 = call-by-ref "?"(reference=w342, "Action"=AlliGator_FLI_Image_Stack_Action."Init", "error in (no error)"=w340, "File Info"=w343) -> (reference out=w341:refnum<vi>, "error out"=w344:errorcluster)  [unwired: 7 in, 3 out]
        }
      }
      n21 = case shown="No Error" w204 {
        selector: w204 -> [w395 w608]
        tunnel: [w379 _] -> w217
        tunnel: w216 -> [w401 _]
        tunnel: w215 -> [w400 _]
        tunnel: [w397 _] -> w214
        tunnel: w213 -> [w396 _]
        tunnel: w209 -> [w359 _]
        tunnel: [w394 _] -> w212
        tunnel: w210 -> [w387 _]
        tunnel: w211 -> [w388 _]
        tunnel: w195 -> [w392 _]
        tunnel: [w355 w608] -> w146
        tunnel: [w376 w607] -> w156
        tunnel: [w380 w606] -> w169
        tunnel: [w358 w605] -> w184
        tunnel: [w357 w604] -> w183
        tunnel: w185 -> [_ w605]
        tunnel: w181 -> [_ w604]
        tunnel: w171 -> [_ w606]
        tunnel: w154 -> [_ w607]
        tunnel: w186 -> [w367 _]
        tunnel: w180 -> [_ w603]
        tunnel: [w381 w603] -> w179
        tunnel: w153 -> [_ w602]
        tunnel: [_ w602] -> w164
        tunnel: w206 -> [w391 _]
        tunnel: w205 -> [w390 _]
        tunnel: w200 -> [w386 w595]
        tunnel: [w384 _] -> w199
        tunnel: w161 -> [_ _]
        tunnel: w198 -> [w383 _]
        tunnel: w174 -> [_ w601]
        tunnel: w177 -> [_ w600]
        tunnel: w194 -> [w370 _]
        tunnel: w197 -> [w371 _]
        tunnel: [w381 w601] -> w172
        tunnel: [w380 w600] -> w175
        tunnel: w148 -> [w378 _]
        tunnel: w152 -> [w368 w599]
        tunnel: [w369 w599] -> w166
        tunnel: w151 -> [_ w598]
        tunnel: w150 -> [_ w597]
        tunnel: [w371 w598] -> w168
        tunnel: [w375 w597] -> w159
        tunnel: w191 -> [w375 _]
        tunnel: [w373 _] -> w190
        tunnel: [w372 _] -> w189
        tunnel: w157 -> [w366 w596]
        tunnel: [w365 w596] -> w188
        tunnel: w187 -> [w361 _]
        tunnel: [w360 _] -> w149
        tunnel: w141 -> [w348 _]
        tunnel: [w347 _] -> w139
        tunnel: [w346 w595] -> w138
        frame No Error {
          w403 = 0  # Current Gate
          w404 = TRUE  # Init?
          w402 = 0  # # created images
          # "Index 2 images are only used for dual-gate datasets"
          # "Images 2"
          # "Bkgd Images 2"
          # "Buffer Images 2"
          # "Images 1"
          # "Bkgd Images 1"
          # "Buffer Images 1"
          n22 = call "Pseudo-random (Time-based) String.vi"("Length (10)"=u32 10) -> ("result string"=w389:string)  [unwired: 9 in, 1 out]
          n23 = call "Embedded Progress Bar Q.vi"("Progress Bar Queue Name"="AlliGator Progress Bar Q") -> ("Progress Bar Queue"=w352:refnum<queue>)  [unwired: 6 in]
          n24 = call "Send Embedded Progress Bar Update.vi"("Max Iterations N"=w348, "Current Iteration i (i or -1: standard or || iteration; 0 or -2: first standard or || iteration)"=-2 ("Current Iteration i (i or -1: standard or || iteration; 0 or -2: first standard or || iteration)"), "Progress Bar Queue in"=w352) -> ("Progress Bar Queue out"=w351:refnum<queue>)  [unwired: 7 in, 1 out]
          n25 = while {
            tunnel: w401 -> [w458]
            shift-right: [w439] -> w393
            shift-left: w395 -> [w447]
            shift-right: [w450] -> _
            shift-left: w404 -> [w460]
            shift-right: [w437] -> w376
            shift-left: w403 -> [w459]
            shift-right: [w448] -> w379
            shift-left: w402 -> [w455]
            shift-right: [w453] -> _
            shift-left: _ -> [w427]
            tunnel: w400 -> [w466]
            tunnel: w389 -> [w462]
            tunnel: [w449] -> w399 mode=indexing
            shift-right: [w452] -> _
            shift-left: _ -> [w426]
            shift-right: [w451] -> w381
            shift-left: _ -> [w463]
            tunnel: w367 -> [w464]
            tunnel: w396 -> [w456]
            tunnel: [w465] -> w394
            tunnel: w392 -> [w445]
            tunnel: w391 -> [w444]
            tunnel: w390 -> [w443]
            tunnel: w386 -> [w442]
            tunnel: [w441] -> w385 mode=indexing
            tunnel: w383 -> [w436]
            shift-right: [w428] -> _
            shift-left: _ -> [w425]
            shift-right: [w430] -> _
            shift-left: _ -> [w424]
            shift-right: [w429] -> w380
            shift-left: _ -> [w435]
            tunnel: w370 -> [w433]
            tunnel: [w431] -> w382
            tunnel: w378 -> [w420]
            tunnel: [w419] -> w374 mode=indexing if=w418
            tunnel: [w417] -> w360
            tunnel: w351 -> [w415]
            tunnel: [w414] -> w349
            tunnel: [w412] -> w347
            tunnel: [w411] -> w346
            i -> [w446]
            stop <- w413 stop-if-true
            n26 = Greater Or Equal?(x=w446, y=w445) -> (x >= y?=w421:bool)
            n27 = case shown="False" w460 {
              tunnel: w464 -> [w583 w590]
              tunnel: [w583 w590] -> w431
              tunnel: w427 -> [_ w587]
              tunnel: w426 -> [_ w588]
              tunnel: w463 -> [w582 _]
              tunnel: [w582 w589] -> w461
              tunnel: w425 -> [_ w586]
              tunnel: w424 -> [_ w584]
              tunnel: [w581 w585] -> w434
              tunnel: w435 -> [w581 _]
              frame False {
              }
              frame True {
                # "Select which images to update"
                n28 = case shown="False" w590 {
                  tunnel: [w592 w594] -> w589
                  tunnel: w588 -> [_ w594]
                  tunnel: w587 -> [w592 _]
                  tunnel: w586 -> [w591 _]
                  tunnel: [w591 w593] -> w585
                  tunnel: w584 -> [_ w593]
                  frame False {
                  }
                  frame True {
                  }
                }
              }
            }
            n29 = Search 1D Array(1D array=w466, element=w446) -> (index of element=w457:i32)  [unwired: 1 in]
            n30 = Greater Or Equal To 0?(x=w457) -> (x >= 0?=w423:bool)
            n31 = call "Send Embedded Progress Bar Update.vi"("Current Iteration i (i or -1: standard or || iteration; 0 or -2: first standard or || iteration)"=-1 ("Current Iteration i (-1: || iteration, -2: first || iteration)"), "Progress Bar Queue in"=w415) -> ("Progress Bar Queue out"=w414:refnum<queue>)  [unwired: 8 in, 1 out]
            n32 = Compound Arithmetic op=AND(w420, w423) -> (w422:bool)
            n33 = case shown="False" w422 {
              tunnel: w447 -> [w546 w580]
              tunnel: w456 -> [w520 _]
              tunnel: w458 -> [w554 _]
              tunnel: w460 -> [w519 w578]
              tunnel: [w510 w578] -> w450
              tunnel: w459 -> [w522 w575]
              tunnel: [w541 w576] -> w454
              tunnel: w455 -> [w552 w579]
              tunnel: [w553 w579] -> w448
              tunnel: [w544 w580] -> w440
              tunnel: w462 -> [w529 _]
              tunnel: [w551 _] -> w449
              tunnel: w431 -> [w511 _]
              tunnel: w446 -> [w549 _]
              tunnel: w461 -> [w535 w576]
              tunnel: w442 -> [w548 w577]
              tunnel: [w542 _] -> w441
              tunnel: [w540 w577] -> w438
              tunnel: [w509 w575] -> w437
              tunnel: w436 -> [w525 _]
              tunnel: w434 -> [w532 w574]
              tunnel: w433 -> [w521 _]
              tunnel: [w512 w574] -> w432
              tunnel: [w508 _] -> w419
              tunnel: [w505 _] -> w418
              frame True {
                n34 = call "High Resolution Timing.vi"("Error In"=w546) -> ("elapsed (relative) seconds"=w543:dbl, "Error Out"=w517:errorcluster)  [unwired: 16 in, 1 out]
                n35 = Index Array(array=w554, index=w549) -> (element=w531:string)
                n36 = call-by-ref "?"(reference=w548, error in=w517, "Action"=AlliGator_FLI_Image_Stack_Action."Get Image", 8:"error in (no error)"=w517, "Gate Index"=w549) -> (reference out=w540:refnum<vi>, error out=w516:errorcluster, 0:"error out"=w518:errorcluster, "Data 2"=w534:sgl[][], "Data 1"=w547:sgl[][])  [unwired: 6 in]
                n37 = Concatenate Strings("1" ("string"), w529) -> (w530:string)
                n38 = call "AlliGator Create Gate Image v2.vi"("Dataset Images in"=w535, "Init?"=w519, "Prefix"=w530, "Current Gate"=w522, "Gate Name"=w531, "error in (no error)"=w517, "Image Characteristics"=w520, "Background Dataset"=w511) -> ("Init?"=w510:bool, "Dataset Images out"=w536:T25, "New Gate Image Refnum"=w537:T24, "Buffer Image available?"=w524:bool, "Number of Created Images"=w538:i32, "error out"=w515:errorcluster)  [unwired: 2 in]
                n39 = Merge Errors(w516, w518) -> (w513:errorcluster)
                n40 = Merge Errors(w515, w513) -> (w514:errorcluster)
                n41 = Concatenate Strings("2" ("string"), w529) -> (w527:string)
                n42 = case shown="False" w521 {
                  tunnel: w534 -> [_ w573]
                  tunnel: [w556 w572] -> w533
                  tunnel: w532 -> [w555 w571]
                  tunnel: w531 -> [_ w570]
                  tunnel: w513 -> [w556 w569]
                  tunnel: w519 -> [_ w568]
                  tunnel: w527 -> [_ w567]
                  tunnel: w525 -> [_ w564]
                  tunnel: [_ w562] -> w523
                  tunnel: w522 -> [_ w560]
                  tunnel: w520 -> [_ w559]
                  tunnel: [w555 w558] -> w512
                  tunnel: w511 -> [_ w557]
                  frame False {
                    # "Single-Channel Dataset"
                  }
                  frame True {
                    # "Dual-Channel Dataset"
                    n43 = call "AlliGator Create Gate Image v2.vi"("Dataset Images in"=w571, "Init?"=w568, "Prefix"=w567, "Current Gate"=w560, "Gate Name"=w570, "error in (no error)"=w569, "Image Characteristics"=w559, "Background Dataset"=w557) -> ("Init?"=w563:bool, "Dataset Images out"=w566:T25, "New Gate Image Refnum"=w565:T24, "Number of Created Images"=w562:i32, "error out"=w561:errorcluster)  [unwired: 2 in, 1 out]
                    n44 = call "AlliGator Image Pre-processing.vi"("Image Pre-Processing Parameters"=w564, "Data"=w573, "Buffer Image available?"=w563, "error in (no error)"=w561, "Current Gate"=w560, "Refnum in"=w565, "Dataset Images in"=w566) -> ("error out"=w572:errorcluster, "Dataset Images out"=w558:T25)  [unwired: 3 out]
                  }
                }
                n45 = Compound Arithmetic op=ADD(w523, w538, w552) -> (w553:i32)
                n46 = call "AlliGator Image Pre-processing.vi"("Image Pre-Processing Parameters"=w525, "Data"=w547, "Buffer Image available?"=w524, "error in (no error)"=w514, "Current Gate"=w522, "Refnum in"=w537, "Dataset Images in"=w536) -> ("error out"=w545:errorcluster, "Current Gate (dup)"=w539:i32, "# Replacements"=w551:i32, "Dataset Images out"=w541:T25, "Image Resolution"=w508:cluster{"X Resolution":i32, "Y Resolution":i32})
                n47 = Merge Errors(w545, w533) -> (w507:errorcluster)
                n48 = Unbundle By Name(w507) -> ("status"=w506:bool)
                n49 = Increment(x=w539) -> (x+1=w509:i32)
                n50 = Not(x=w506) -> (.not. x?=w505:bool)
                n51 = call "High Resolution Timing.vi"("relative seconds (NaN)"=w543, "Error In"=w507) -> ("elapsed (relative) seconds"=w542:dbl, "Error Out"=w544:errorcluster)  [unwired: 15 in, 1 out]
              }
              frame False {
                # "this gate mage is not used (e.g. skipped)\nor we are dealing with an already loaded background dataset"
              }
            }
            n52 = global read "AlliGator Abort.vi" "Abort?"() -> (w412:bool)
            n53 = Compound Arithmetic op=OR(w421, w412) -> (w413:bool)
            n54 = Compound Arithmetic op=AND(w420, w421) -> (w417:bool)
            n55 = case shown="False" w417 {
              tunnel: [_ w496] -> w465
              tunnel: w454 -> [w472 w495]
              tunnel: [w474 w494] -> w453
              tunnel: [w473 w493] -> w452
              tunnel: [w472 w492] -> w451
              tunnel: w444 -> [_ w491]
              tunnel: w443 -> [_ w490]
              tunnel: w440 -> [w468 w488]
              tunnel: [w468 w487] -> w439
              tunnel: w438 -> [w467 w475]
              tunnel: w437 -> [_ w486]
              tunnel: w432 -> [w469 w485]
              tunnel: w431 -> [_ w483]
              tunnel: [w470 w482] -> w430
              tunnel: [w469 w481] -> w429
              tunnel: [w471 w480] -> w428
              tunnel: w427 -> [w474 w479]
              tunnel: w426 -> [w473 w478]
              tunnel: w425 -> [w471 w477]
              tunnel: w424 -> [w470 w476]
              tunnel: [w467 w475] -> w411
              frame False {
                # "if not done loading the gates, or \nnot reloading the background dataset"
              }
              frame True {
                # "Last step: updates shift register-stored data"
                n56 = call "AlliGator Last Gate Loading.vi"("Dataset Images 1 in"=w495, "Gates across boundaries?"=w490, "Split Index"=w491, "Dataset Images 2 in"=w485, "Current Gate"=w486, "VI in"=w475, "error in (no error)"=w488) -> ("Dataset Images 1 out"=w489:T25, "Dataset Images 2 out"=w484:T25, "# Disposed Images"=w496:i32, "error out"=w487:errorcluster)  [unwired: 5 in]
                n57 = case shown="True" w483 {
                  tunnel: [w500 w503] -> w493
                  tunnel: w489 -> [w499 w503]
                  tunnel: [w499 w504] -> w494
                  tunnel: w479 -> [_ w504]
                  tunnel: w478 -> [w500 _]
                  tunnel: [w499 w503] -> w492
                  tunnel: w484 -> [w498 w502]
                  tunnel: [w497 w502] -> w482
                  tunnel: [w498 w502] -> w481
                  tunnel: [w498 w501] -> w480
                  tunnel: w477 -> [_ w501]
                  tunnel: w476 -> [w497 _]
                  frame False {
                  }
                  frame True {
                  }
                }
              }
            }
          }
          n58 = case shown="True" w367 {
            tunnel: w370 -> [w407 w409]
            tunnel: [w407 w410] -> w369
            tunnel: w368 -> [_ w410]
            tunnel: w366 -> [w406 _]
            tunnel: [w406 w409] -> w365
            tunnel: [AlliGator_Variables_List."Files:Dataset Channel" ("Alligator Variable") AlliGator_Variables_List."Files:Background Dataset Channel" ("Alligator Variable")] -> w362
            frame False {
              # "Dataset"
            }
            frame True {
              # "background"
              # "Bkgd"
            }
          }
          n59 = call "Send Embedded Progress Bar Update.vi"("Stop Progress Bar (F)"=TRUE, "Progress Bar Queue in"=w349) -> ()  [unwired: 8 in, 2 out]
          n60 = Add Array Elements(numeric array=w385) -> (sum=w384:dbl)
          n61 = Add Array Elements(numeric array=w399) -> (sum=w398:i32)
          n62 = call "Get Common Image Resolution.vi"("Array of Image Resolutions"=w374) -> ("Y Resolution"=w372:i32, "X Resolution"=w373:i32)  [unwired: 8 in, 1 out]
          n63 = call "Number of Inf to NaN Conversions String.vi"("# Inf >> NaN"=w398) -> ("# inf >> NaN Conversion Sring"=w397:string)
          n64 = call "AlliGator Update Background File Subtraction Information.vi"("Background subtracted"=w382, "Error In"=w393, "Background Dataset Path"=w359, "Background Pixel Well Capacity"=w387, "Background Pile-up Correction"=w388) -> ("Error Out"=w364:errorcluster)  [unwired: 6 in]
          n65 = call "Alligator Variables Storage.vi"("Get(F)/Set"=TRUE, "AlliGator Variable"=w362, "Error In"=w364, "Data in"=w361) -> ("Error Out"=w356:errorcluster)  [unwired: 5 in, 2 out]
          n66 = call "Get File Name or Folder Name (wo .ext).vi"("error in (no error)"=w356, "input path"=w359) -> ("error out"=w355:errorcluster, "filename without extension"=w357:string, "dup path"=w358:path)  [unwired: 7 in]
        }
        frame Error {
        }
      }
      n67 = case shown="False" w139 {
        tunnel: w186 -> [w268 _]
        tunnel: w185 -> [w267 w327]
        tunnel: w184 -> [w266 _]
        tunnel: w183 -> [w265 _]
        tunnel: [w264 w320] -> w182
        tunnel: w181 -> [w263 w320]
        tunnel: w180 -> [w262 w331]
        tunnel: w179 -> [w261 _]
        tunnel: [w260 w331] -> w178
        tunnel: w177 -> [w259 w329]
        tunnel: [w258 w329] -> w176
        tunnel: w175 -> [w257 _]
        tunnel: w174 -> [w256 w330]
        tunnel: [w255 w330] -> w173
        tunnel: w172 -> [w254 _]
        tunnel: w171 -> [w253 w328]
        tunnel: [w252 w328] -> w170
        tunnel: w169 -> [w251 _]
        tunnel: w168 -> [w250 _]
        tunnel: [w249 w324] -> w167
        tunnel: w166 -> [w248 _]
        tunnel: [w247 w319] -> w165
        tunnel: w164 -> [w246 _]
        tunnel: [w245 w323] -> w163
        tunnel: [w244 w326] -> w162
        tunnel: w161 -> [w243 _]
        tunnel: w160 -> [w242 w326]
        tunnel: w159 -> [w241 _]
        tunnel: [w240 w325] -> w158
        tunnel: w156 -> [w239 _]
        tunnel: [w238 w321] -> w155
        tunnel: w154 -> [w237 w321]
        tunnel: w153 -> [w236 w323]
        tunnel: w152 -> [w235 w319]
        tunnel: w151 -> [w234 w324]
        tunnel: w150 -> [w233 w325]
        tunnel: w136 -> [w232 _]
        tunnel: w137 -> [w231 _]
        tunnel: [w230 w327] -> w147
        tunnel: w146 -> [w222 _]
        tunnel: w145 -> [w229 _]
        tunnel: w144 -> [w219 _]
        tunnel: [w220 w322] -> w143
        tunnel: w133 -> [w228 w322]
        tunnel: [w227 w318] -> w140
        tunnel: w138 -> [_ w315]
        tunnel: w137 -> [w226 _]
        tunnel: w136 -> [w225 _]
        tunnel: w135 -> [w224 _]
        tunnel: w134 -> [w223 _]
        tunnel: w133 -> [w221 _]
        frame False {
          n68 = case shown="False" w268 {
            tunnel: w267 -> [_ w313]
            tunnel: [w288 w313] -> w230
            tunnel: w266 -> [w288 _]
            tunnel: w265 -> [w299 _]
            tunnel: [w299 w312] -> w264
            tunnel: w263 -> [_ w312]
            tunnel: w262 -> [w298 _]
            tunnel: w261 -> [_ w311]
            tunnel: [w298 w311] -> w260
            tunnel: w259 -> [w297 _]
            tunnel: [w297 w310] -> w258
            tunnel: w257 -> [_ w310]
            tunnel: w256 -> [_ w309]
            tunnel: [w296 w309] -> w255
            tunnel: w254 -> [w296 _]
            tunnel: w253 -> [_ w308]
            tunnel: [w295 w308] -> w252
            tunnel: w251 -> [w295 _]
            tunnel: w250 -> [w290 _]
            tunnel: [w290 w303] -> w249
            tunnel: w248 -> [w291 _]
            tunnel: [w291 w304] -> w247
            tunnel: w246 -> [w292 _]
            tunnel: [w292 w305] -> w245
            tunnel: w243 -> [w293 _]
            tunnel: [w293 w306] -> w244
            tunnel: w242 -> [_ w306]
            tunnel: w241 -> [w289 _]
            tunnel: [w289 w302] -> w240
            tunnel: w239 -> [w294 _]
            tunnel: [w294 w307] -> w238
            tunnel: w237 -> [_ w307]
            tunnel: w236 -> [_ w305]
            tunnel: w235 -> [_ w304]
            tunnel: w234 -> [_ w303]
            tunnel: w233 -> [_ w302]
            tunnel: w226 -> [w287 _]
            tunnel: w225 -> [w286 _]
            tunnel: w224 -> [w285 _]
            tunnel: w223 -> [w283 _]
            tunnel: w222 -> [w284 w300]
            tunnel: w221 -> [w281 w301]
            tunnel: [w280 w301] -> w220
            tunnel: [w279 w300] -> w218
            frame False {
              # "Image Dataset"
              n69 = call "AlliGator Update Dataset Series Slide.vi"("Dataset Series Slide Ref"=w283, "Current Time Stamp Ref"=w285, "Error In"=w284, "Path"=w288, "Dataset Series Paths"=w287, "Dataset Series Timestamps"=w286) -> ("Error Out"=w279:errorcluster, "Current Dataset"=w282:i32)  [unwired: 4 in]
              n70 = Select(t=w281, s=w279, f=w282) -> (s? t:f=w280:i32)
            }
            frame True {
              # "Background Dataset"
            }
          }
          n71 = disable-structure shown="Enabled" {
            disable-tunnel: w232 -> [w277 _]
            disable-tunnel: w231 -> [w276 _]
            disable-tunnel: w230 -> [w275 _]
            disable-tunnel: w229 -> [w274 _]
            disable-tunnel: w228 -> [w272 _]
            disable-tunnel: [w271 w278] -> w227
            disable-tunnel: w218 -> [w270 w278]
            disable-tunnel: w219 -> [w269 _]
            frame Disabled {
              n72 = call "AlliGator Update Dataset Series Slide.vi"("Dataset Series Slide Ref"=w269, "Current Time Stamp Ref"=w274, "Error In"=w270, "Path"=w275, "Dataset Series Paths"=w276, "Dataset Series Timestamps"=w277) -> ("Error Out"=w271:errorcluster, "Current Dataset"=w273:i32)  [unwired: 4 in]
              n73 = Select(t=w272, s=w271, f=w273) -> ()  [unwired: 1 out]
            }
            frame Enabled {
            }
          }
        }
        frame True {
          # "loading aborted"
          n74 = xnode "Error Ring"() -> ("error out"=w318:errorcluster)
          n75 = call-by-ref "?"(reference=w315, "Action"=AlliGator_FLI_Image_Stack_Action."Close") -> ("error out"=w314:errorcluster)  [unwired: 9 in, 4 out]
          n76 = call <vilib>:"Clear Errors.vi"("error in (no error)"=w314) -> ()  [unwired: 5 in, 2 out]
          n77 = global write "AlliGator Abort.vi" "Abort?"(FALSE ("Abort?")) -> ()
        }
      }
      n78 = in-place-cluster #2("Current Dataset"=w143, "Dual-Channel Background Dataset"=w188, "# Gates"=w155, "Background Dataset Images 1"=w178, "Current Dataset Images 1"=w173, "Background Dataset Images 2"=w176, "Current Dataset Images 2"=w170, "[Time-Series Timestamps]"=w136, "[Time-Series Paths]"=w137, "Single Data Point Path"=w147, "Current Folder"=w182, "Single Dataset Type"=w162, "I/m/phi Dataset.I/m/phi Dataset?"=w163, "Dual-Channel Dataset"=w165, "Channel Arithmetic"=w167, "Selected Channel Name"=w158) -> (w119:T23)
      n79 = property class="Str"(reference=w208, error in=w140, "Value"=w182) -> (error out=w207:errorcluster)  [unwired: 1 out]
    }
    n80 = in-place-dvr #1(w119) -> (→"Data Value Reference out":refnum<data-value>)  [unwired: 1 out]
  }
  "# Disposed Images" <- w86
  "# created images" <- w85
  "Dual-Channel Dataset" <- w33
  n81 = call "AlliGator Get ICCD Information.vi"("Y Resolution"=w3, "X Resolution"=w4, "Error In"=w9, "Y Software Binning"=w5, "X Software Binning"=w6, "File Info"=w11) -> ("Error Out"=w8:errorcluster, "ICCD-specific Information"=w10:T59)  [unwired: 4 in]
  n82 = case shown="False" w20 {
    tunnel: w89 -> [_ w650]
    tunnel: w79 -> [_ w648]
    tunnel: w78 -> [_ w647]
    tunnel: w76 -> [_ w646]
    tunnel: w75 -> [_ w643]
    tunnel: w74 -> [_ w642]
    tunnel: w73 -> [_ w641]
    tunnel: w72 -> [_ w640]
    tunnel: w66 -> [_ w639]
    tunnel: w65 -> [_ w638]
    tunnel: [w610 w637] -> w57
    tunnel: w52 -> [_ w636]
    tunnel: w48 -> [_ w632]
    tunnel: [w609 w631] -> w47
    tunnel: w7 -> [_ w630]
    tunnel: "selected path" -> [_ w629]
    tunnel: w44 -> [_ w628]
    tunnel: w6 -> [_ w627]
    tunnel: w5 -> [_ w626]
    tunnel: w32 -> [_ w625]
    tunnel: w30 -> [_ w624]
    tunnel: w29 -> [_ w623]
    tunnel: w4 -> [_ w622]
    tunnel: w3 -> [_ w621]
    tunnel: w27 -> [_ w620]
    tunnel: w26 -> [_ w619]
    tunnel: w24 -> [_ w618]
    tunnel: "Metadata" -> [_ w617]
    tunnel: "Data Description" -> [_ w616]
    tunnel: w21 -> [_ w615]
    tunnel: w8 -> [w610 w614]
    tunnel: w19 -> [w611 _]
    tunnel: w10 -> [_ w613]
    frame False {
      # "can be False if error or background file is unchanged"
      n83 = case shown="True" w611 {
        tunnel: ["Background Dataset unchanged (and not reloaded)" _] -> w609
        frame False {
          # "Background Dataset already loaded"
        }
        frame True {
          # "FLI Dataset & Error"
        }
      }
    }
    frame True {
      n84 = Bundle By Name(cluster=T60 {"Nanotime Gate Separation"=0.0, "Gate Width"=0.0, "Laser Period"=0.0, "Data Description"="", "# Pixel X"=0, "# Pixel Y"=0, "Gates to Use"={"Start"=0, "End"=0}, "Gate Step"=0, "SYNC Period"=0.0, "X Binning"=0, "Y Binning"=0, "Gates to"=FALSE, "Metadata"="", "Gate Image Exposure"=0.0, "Gate Image Integration"=0.0, "Macrotime Gate Separation"=0.0, "ICCD-specific Information"={"V MCP"=0.0, "X Hardware Binning"=0.0, "Y Hardware Binning"=0.0, "Gate Image Integration"=0.0, "Laser Power"=0.0}}, "X Binning"=w627, "Y Binning"=w626, "Gates to Use"=w623, "Gates to"=w639, "Nanotime Gate Separation"=w643, "Gate Width"=w646, "Laser Period"=w641, "# Pixel X"=w622, "# Pixel Y"=w621, "Gate Step"=w638, "Data Description"=w616, "SYNC Period"=w642, "Metadata"=w617, "Gate Image Exposure"=w620, "Gate Image Integration"=w619, "Macrotime Gate Separation"=w618, "ICCD-specific Information"=w613) -> (w634:T60)
      n85 = call "AlliGator Update Loaded Dataset Info.vi"("Image Loading Options"=w625, "Background File?"=w640, "Pile-up Correction"=w628, "error in (no error)"=w614, "After Loading Dataset Information"=w634, "# Gates"=w615, "Pixel Well Capacity"=w630) -> ("Error Out"=w635:errorcluster)  [unwired: 4 in]
      n86 = call "High Resolution Timing.vi"("relative seconds (NaN)"=w650, "Error In"=w635) -> ("elapsed (relative) seconds"=w645:dbl, "Error Out"=w644:errorcluster)  [unwired: 15 in, 1 out]
      n87 = Format Into String(format string="%s loaded: %s\n%s%s%s\n# Gates: %d\nLoad time: %#g s\nConversion time: %#g s\n", error in=w644, w647, w629, w632, w636, w624, w615, w645, w648) -> (resulting string=w631:string, error out=w637:errorcluster)  [unwired: 1 in]
    }
  }
  "error out" <- w57
  "Message" <- w47
  n88 = call "Set Slide Range.vi"("Max"=w21, "error in (no error)"=w9, "Slide in"=w56) -> ("error out"=w59:errorcluster)  [unwired: 8 in]
  n89 = Merge Errors(w59, w60) -> (w58:errorcluster)
  n90 = call "Tiny Clear Error.vi"("Error In"=w58) -> ()  [unwired: 8 in, 1 out]
